vi "Master-vi_v1_9_0.vi"() -> ()   [LabVIEW 2024]
uses:
  QMH-Architecture/UI-Controls/UI State.ctl
  QMH-Architecture/support/Control/Waveform Data Constant.ctl
  QMH-Architecture/support/Control/Array Data Constant.ctl
  QMH-Architecture/Aborts/Abort Parameters.ctl
  QMH-Architecture/support/Control/Control Data Constant.ctl
  QMH-Architecture/Sequence/Sequence Structure.ctl
  QMH-Architecture/support/Control/BBControl Parameters.ctl
  QMH-Architecture/Display/Global 1.vi
  <vilib>/Utility/error.llb/Error Cluster From Error Code.vi
  QMH-Architecture/Globals.vi
  <vilib>/ErrorRing/Error Ring.xnode
  QMH-Architecture/support/User Event - Stop/User Event - Stop.lvlib
  QMH-Architecture/support/Message Queue/Message Queue.lvlib
panel:
  out "Total Physical Memory":u64 format="%.1p"
  out "Memory Allocated For LabVIEW":u64 format="%.1p"
  out "Free Physical Memory":u64 format="%.1p"
  out "UI Elements":i32
  out "Acquisition Elements":i32
  out "Logging Elements":i32
  out "Controls Elements":i32
  out "Sequence Elements":i32
  out "Aborts Elements":i32
  out "Processed Data":i32
  out "Unprocessed Data":i32
  out "Controls Iteration Clock":u32
  out "Acquisition Iteration Clock":u32
  out "Processing_Logging Iteration Clock":u32
  out "Sequencing Iteration Clock":u32
  out "Aborts Iteration Clock":u32
  in  "System Monitor":bool
  in  "Control Monitor":bool
  out "Network Stream Clock":u32
  out "NetworkStream Elements":i32
  out "Waveform Chart":i16[](graph)
  in  "Graph Display":bool
  out "Status":T1(array[cluster]) {"Status Timestamp" format="%<%H:%M:%S%3u>T"}
  out "Timestamp":timestamp format="%<%H:%M:%S%3u>T"
  in  "Load Name":bool
  in  "File name":string
  out "Display-Loop Iteration Clock (ms)":u32
  in  "Status clear":bool
  out "Logging Status":bool
  in  "Exit Button":bool
  in  "Stop Button":bool
  in  "Data log":bool
  # "User Interface"
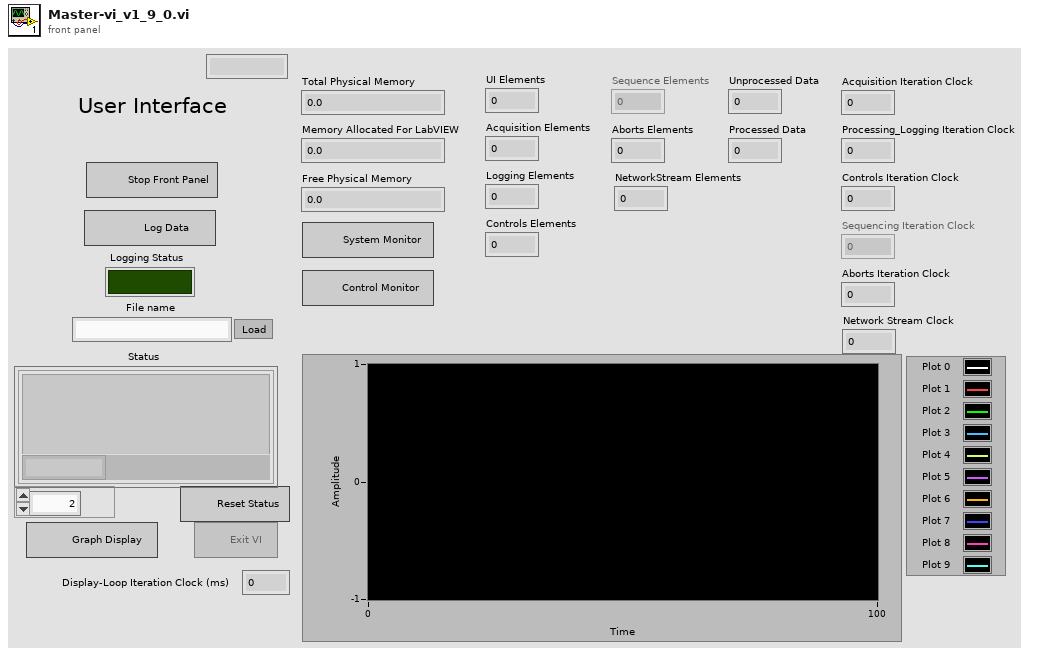
[diagram p1: front panel]
types:
  T1 = cluster{"Status":string, "Status Timestamp":timestamp}[]
  T2 = typedef "BBControl Parameters.ctl" = cluster{"Sequence Delay (s)":dbl, "Sequence Duration (s)":dbl, "BBControl Criteria":cluster{"Channel Name":i32, "Comparison":u16, "Set":dbl, "Enabled":bool, "Valve Name":i32, "Upper":dbl, "Lower":dbl}[]}
  T3 = typedef "Sequence Structure.ctl" = cluster{"Sequence Controller":cluster{"Time (s)":dbl, "Enabled":bool, "Valve":u16[]}[], "Sequence Delay":dbl, "Sequence Duration":dbl}
  T4 = typedef "Control Data Constant.ctl" = cluster{"Time (utc)":ext, "Data Out":cluster{"DO":bool[], "Module Number":string}[]}
  T5 = typedef "Abort Parameters.ctl" = cluster{"Sequence Delay (s)":dbl, "Sequence Duration (s)":dbl, "Abort Criteria":cluster{"Channel Name\n":enum16{"[0]", "[1]", "[2]", "[3]", "[4]", "[5]", "[6]", "[7]", "[8]", "[9]", "[10]", "[11]", "[12]", "[13]", "[14]", "[15]", "[16]", "[17]", "[18]", "[19]", "[20]", "[21]", "[22]", "[23]", "[24]", "[25]", "[26]", "[27]", "[28]", "[29]", "[30]", "[31]", "[32]", "[33]", "[34]", "[35]", "[36]", "[37]", "[38]", "[39]", "[40]", "[41]", "[42]", "[43]", "[44]", "[45]", "[46]", "[47]", "[48]", "[49]"}, "Comparison\n":u16, "Threshold":dbl, "Time on (s)":dbl, "Time off (s)":dbl, "Enabled":bool}[]}
  T6 = typedef "Array Data Constant.ctl" = cluster{"AI":dbl[], "TC":dbl[], "BC":dbl[], "DI":dbl[], "t (UTC)":dbl}
  T7 = typedef "Waveform Data Constant.ctl" = cluster{"AI":waveform(dbl)[], "TC":waveform(dbl)[], "BC":waveform(dbl)[], "DI":digitalwaveform[], "DI2":digitalwaveform[]}
  T8 = typedef "UI State.ctl" = enum16{"Idle", "Acquiring", "Logging", "Waiting for Exit", "Waiting for Exit (Acq Stopped)", "Waiting for Exit (Log Stopped)", "Waiting for Stop", "Waiting for Stop (Acq Stopped)", "Waiting for Stop (Log Stopped)"}
  T9 = typedef "Message Queue.lvlib/All Message Queues.ctl" = cluster{"UI":refnum<queue>, "Acquisition":refnum<queue>, "Logging":refnum<queue>, "Controls":refnum<queue>, "Sequence":refnum<queue>, "Aborts":refnum<queue>, "Network Streams":refnum<queue>}
  T10 = cluster{"Status":string, "Status Timestamp":timestamp}
  T11 = typedef "DAQmx Configuration.ctl" = cluster{"ai DAQmx Cluster":cluster{"ai PXIe Task Name":string[], "input terminal configuration":i32[]}, "bc DAQmx Cluster":cluster{"bc PXIe Task Name":string[], "Scaling Information":cluster{"first electrical value":dbl, "second electrical value":dbl, "electrical units":i32, "first physical value":dbl, "second physical value":dbl, "physical units":i32}[], "Bridge Information":cluster{"bridge configuration":i32, "voltage excitation source":i32, "voltage excitation value":dbl, "nominal bridge resistance":dbl}[]}, "tc DAQmx Cluster":cluster{"tc PXIe Task Name":string[], "Thermocouple Type":i32[], "Units":i32[]}, "di DAQmx Cluster":cluster{"di PXIe Task Name":string[]}, "do DAQmx Cluster":cluster{"do PXIe Task Name":string[]}, "ao DAQmx Cluster":cluster{"ao PXIe Task Name":string[]}}
  T12 = typedef "StreamCluster_TypeDef.ctl" = cluster{"DAQ":cluster{"ManagmentRate_Hz":i32, "StreamRate_Hz":i32, "StreamRate_ms":i32, "ManagmentRate_ms":i32, "refDesArray":cluster{"refDes-s":string[], "Module Number":string}[]}, "Modules":cluster{"Slot ID":i32, "Model Number":string, "Sample Rate s/S (Hz)":dbl, "Sensors":cluster{"refDes":string, "serialNumber":string, "modelNumber":string, "units":string, "balance":dbl, "sensitivity":dbl, "type":string, "inputTerminalConfiguration":string, "channelNumber":string, "taskName":string, "bridgeConfiguration":string, "excitationVoltage":dbl, "voltageExcitationSource":string, "nominalBridgeResistance":dbl, "firstElectricalValue":dbl, "secondElectricalValue":dbl, "firstPhysicalValue":dbl, "secondPhysicalValue":dbl, "electricalUnits":string}[]}[]}
  T13 = typedef "Calibration Configuration.ctl" = cluster{"ai Calibration Slope":dbl[], "ai Calibration Offset":dbl[], "ai Sensor Names ":string[], "tc Sensor Names":string[], "di Sensor Names":string[], "do Sensor Names":string[], "bc Sensor Names":string[], "ai Sensor Units":string[], "tc Sensor Units":string[], "bc Sensor Units":string[]}
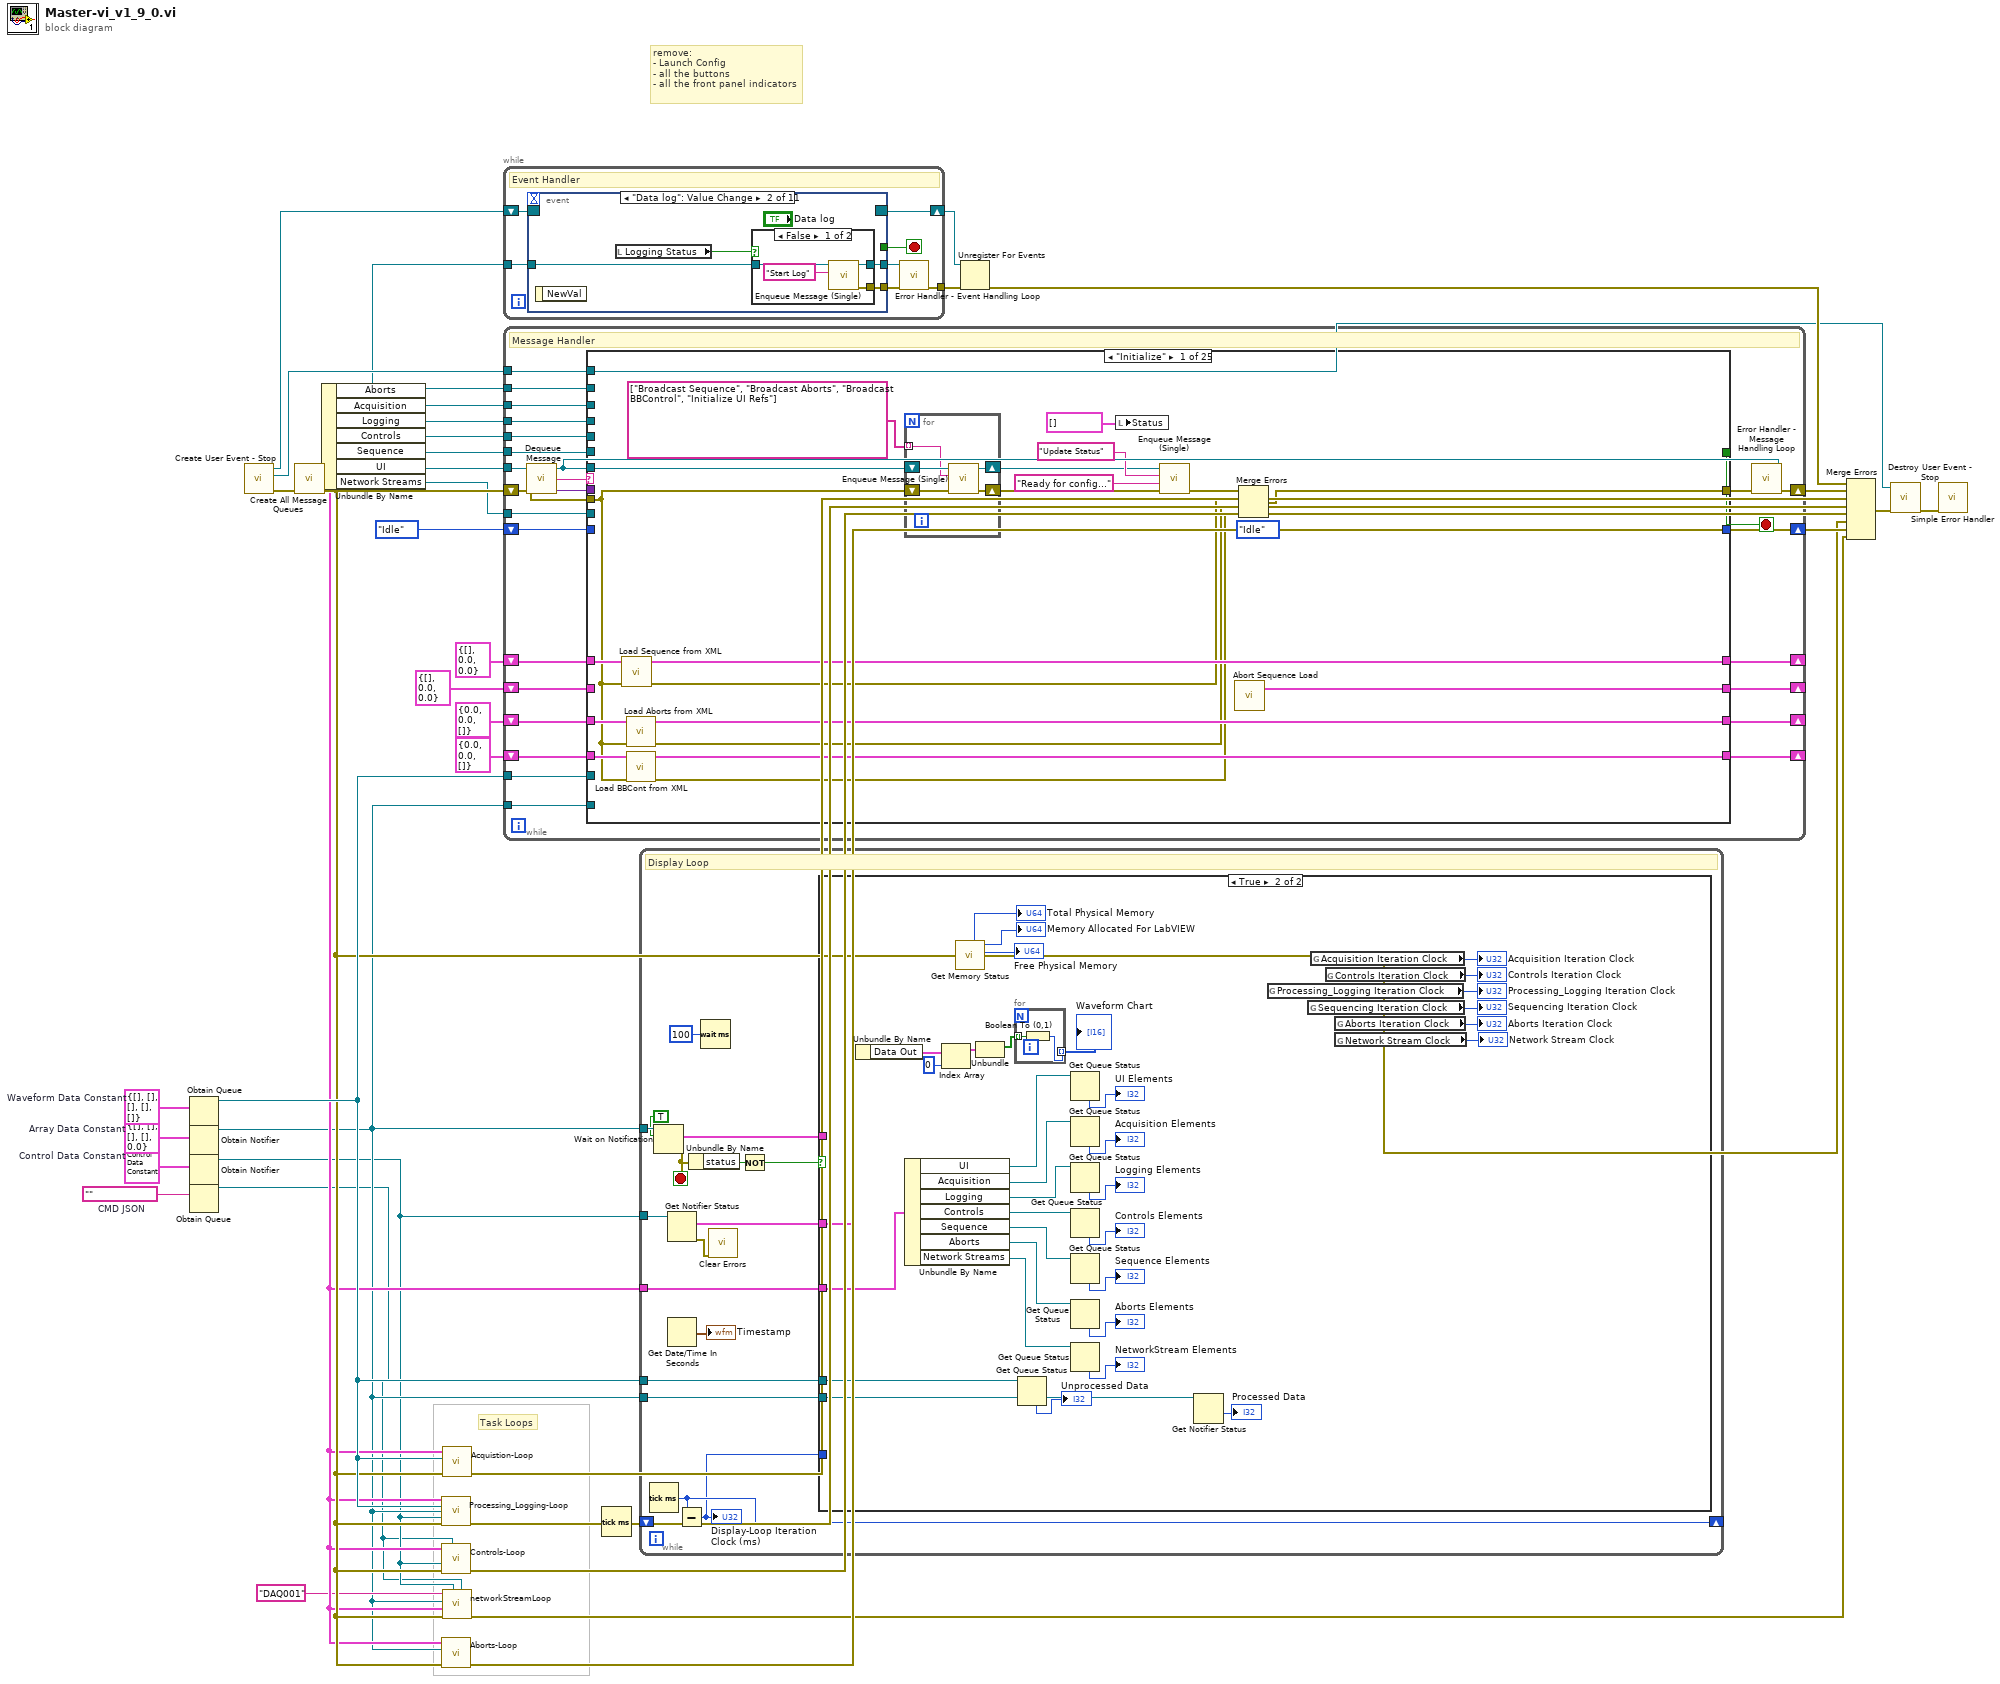
[diagram p0: block diagram]
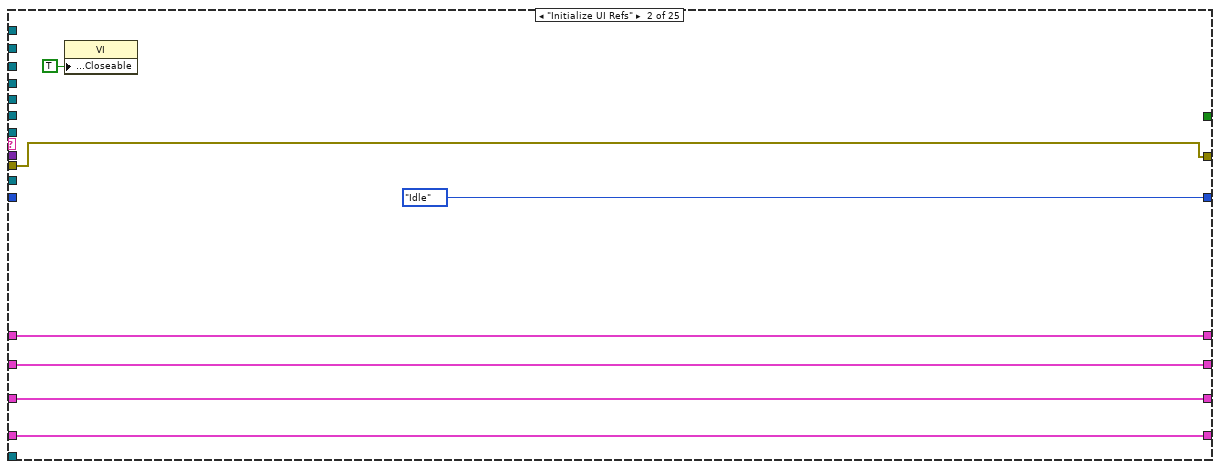
[diagram p3: hidden frame]
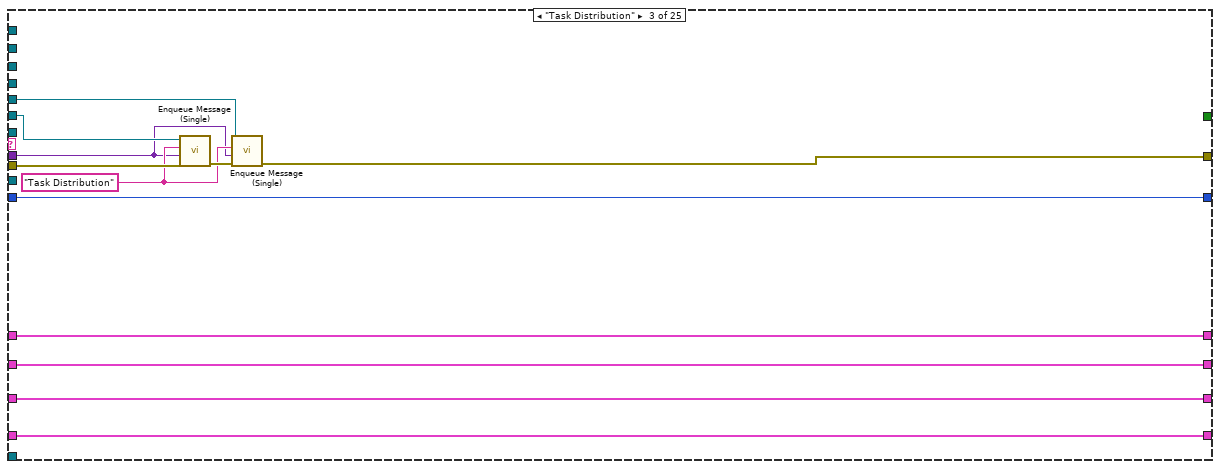
[diagram p4: hidden frame]
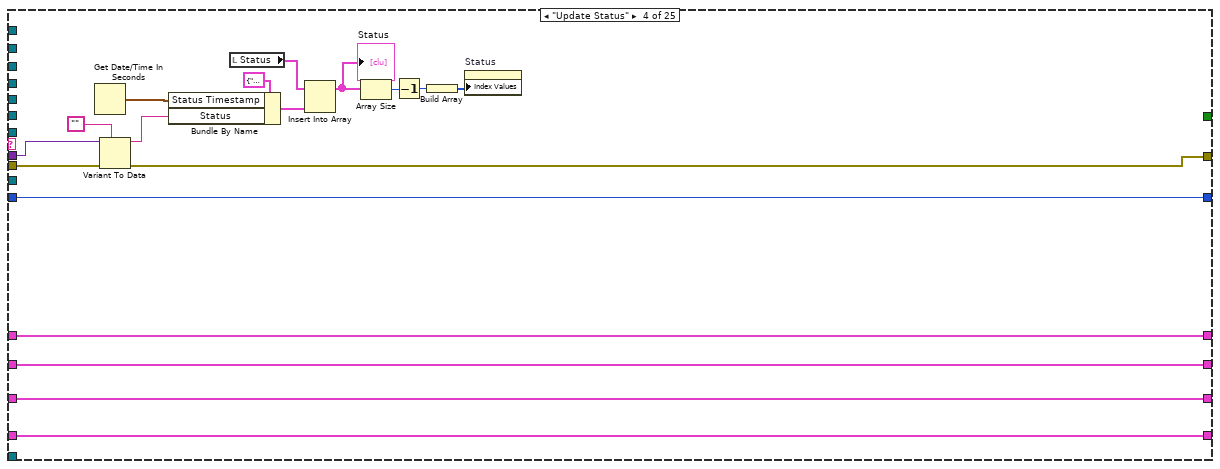
[diagram p5: hidden frame]
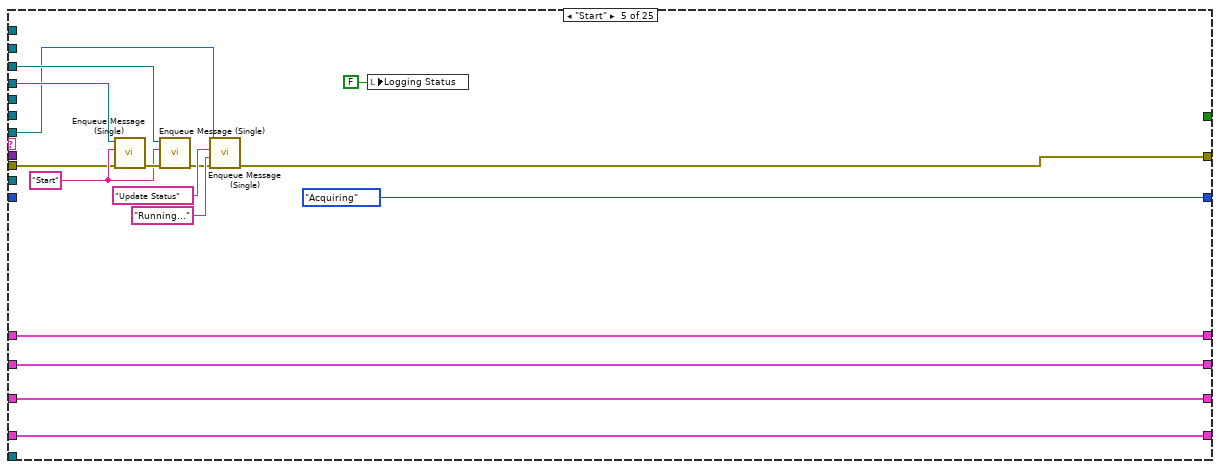
[diagram p6: hidden frame]
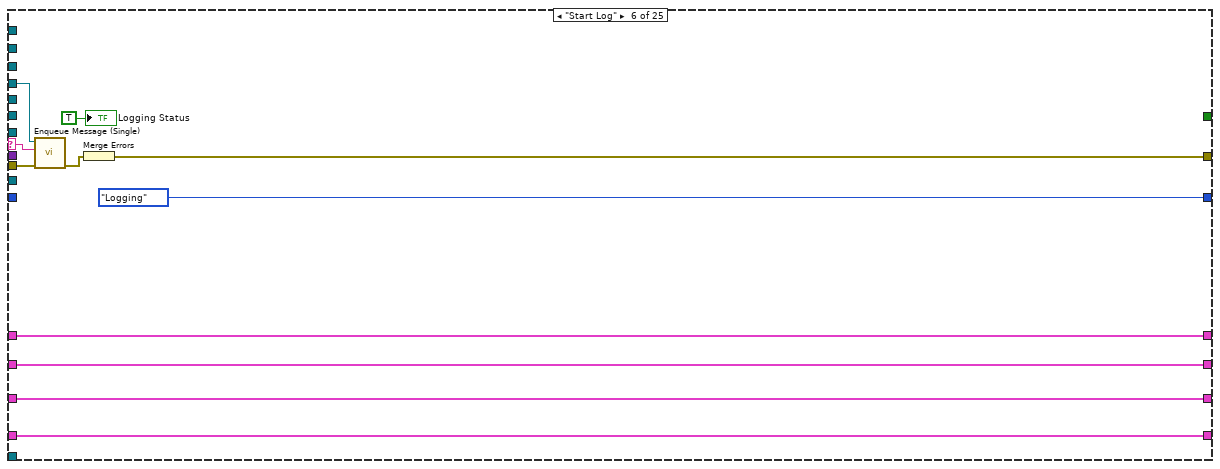
[diagram p7: hidden frame]
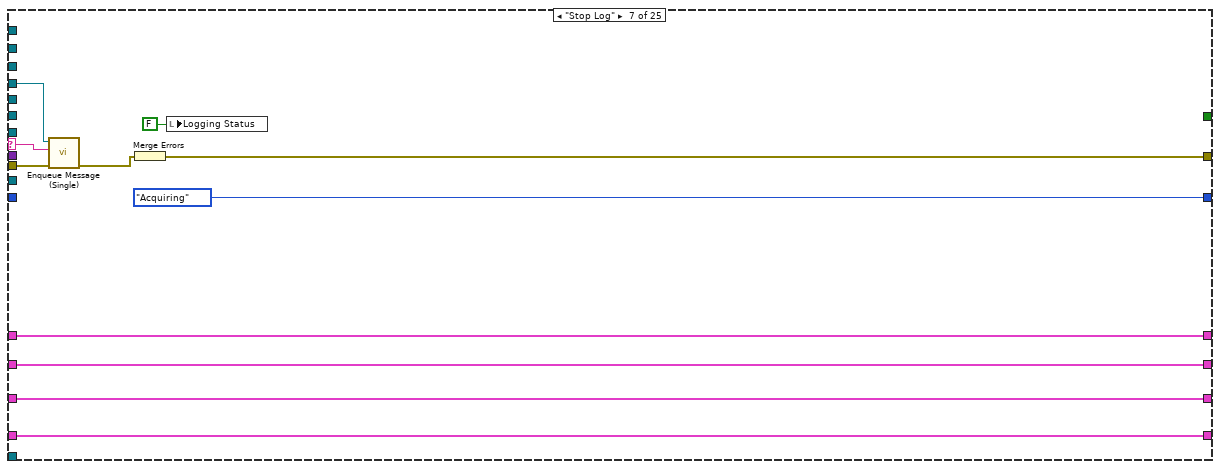
[diagram p8: hidden frame]
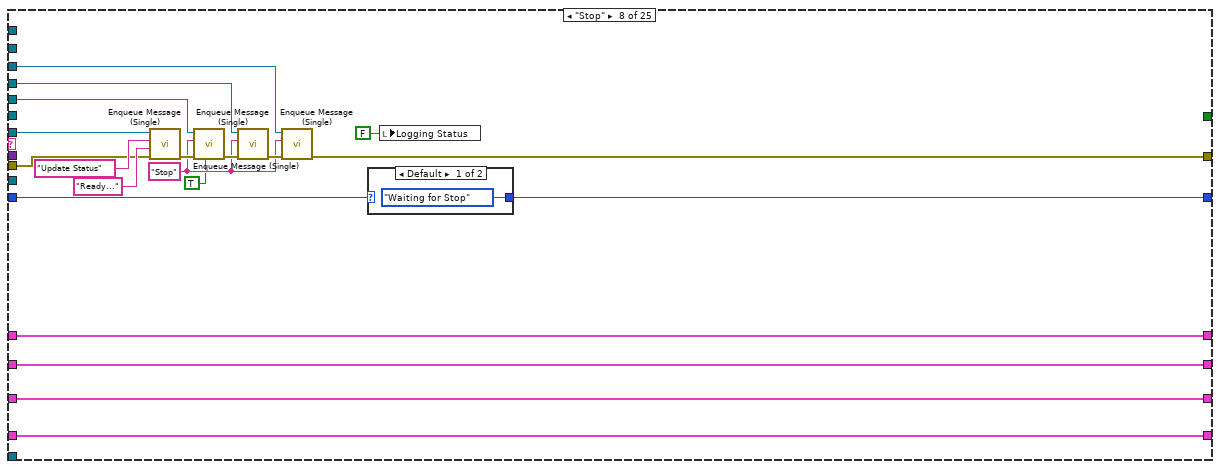
[diagram p9: hidden frame]
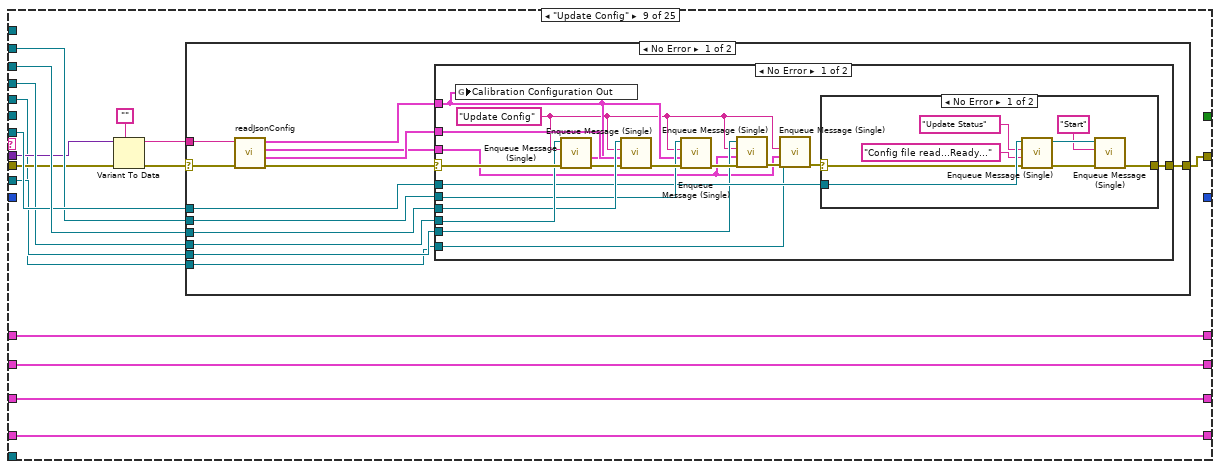
[diagram p11: hidden frame]
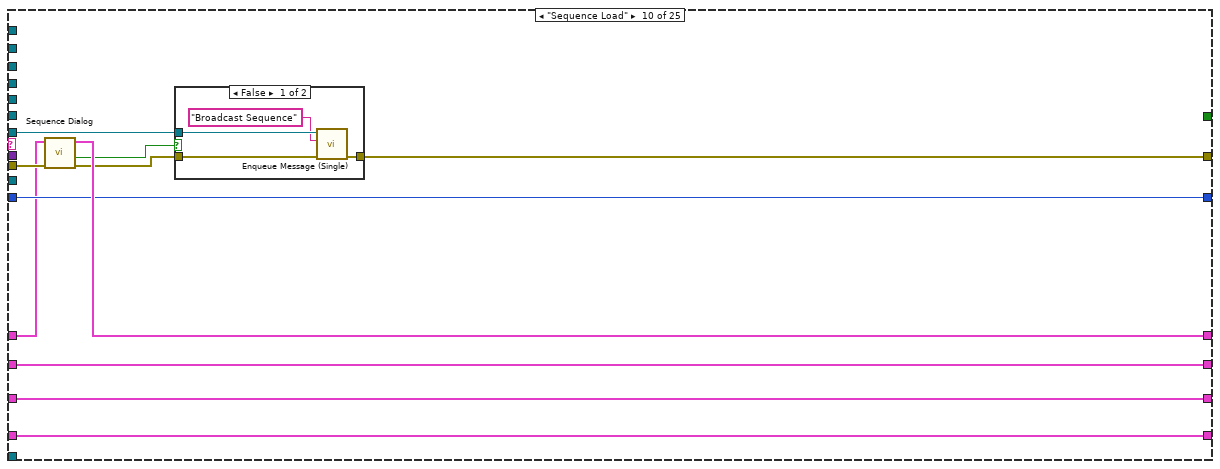
[diagram p15: hidden frame]
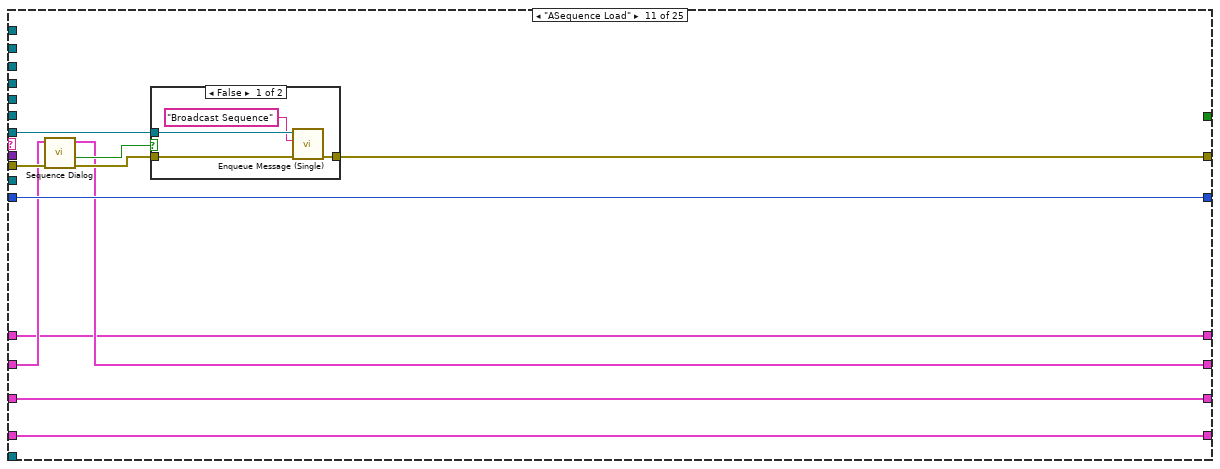
[diagram p17: hidden frame]
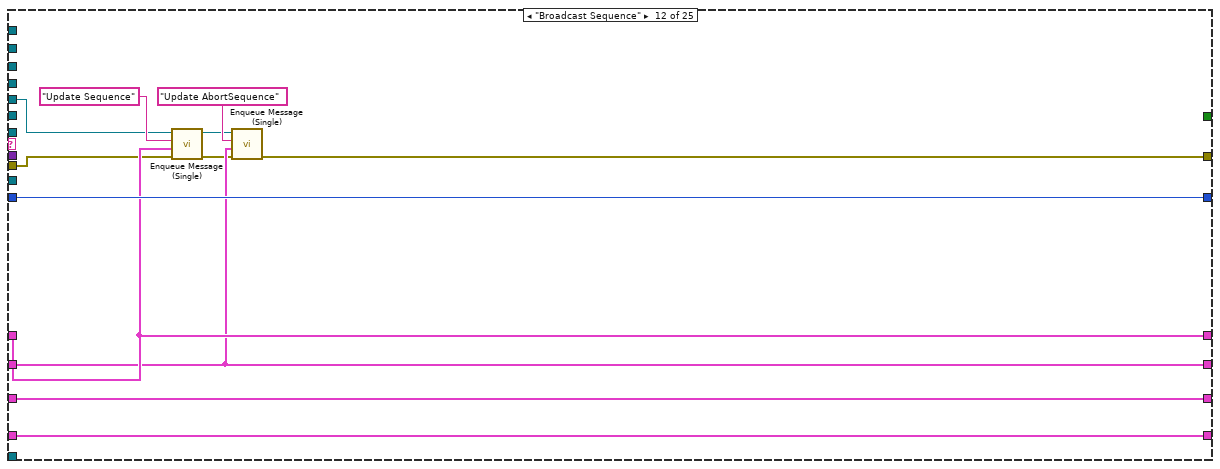
[diagram p19: hidden frame]
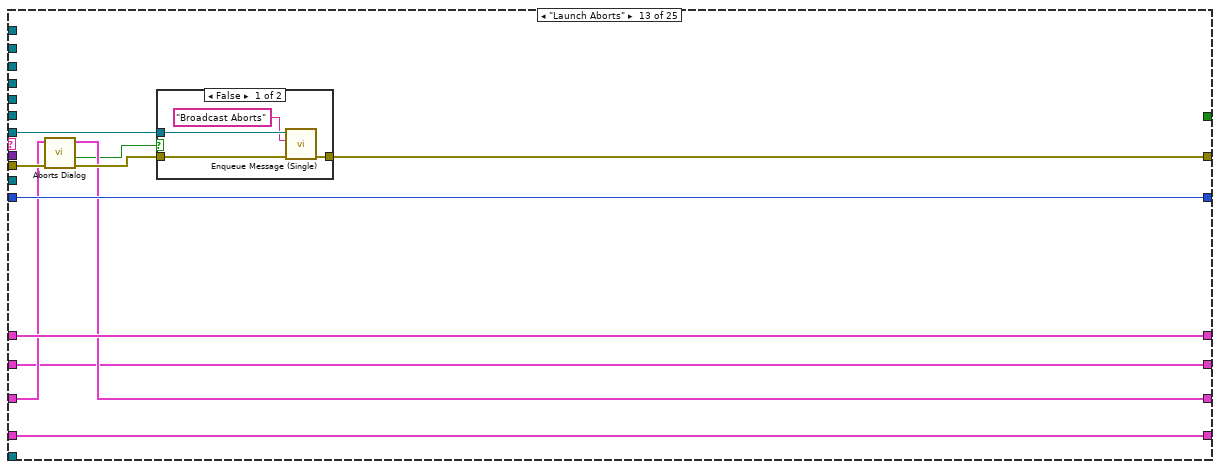
[diagram p20: hidden frame]
diagram:
  w2 = ""  # CMD JSON
  w12 = T4 {"Time (utc)"=0.0, "Data Out"=[]}  # Control Data Constant
  w19 = T6 {"AI"=[], "TC"=[], "BC"=[], "DI"=[], "t (UTC)"=0.0}  # Array Data Constant
  w20 = T7 {"AI"=[], "TC"=[], "BC"=[], "DI"=[], "DI2"=[]}  # Waveform Data Constant
  # "remove:\n- Launch Config\n- all the buttons\n- all the front panel indicators"
  # "Task Loops"
  n1 = Obtain Queue(element data type=w20) -> (queue out=w13:refnum<queue>)  [unwired: 4 in, 2 out]
  n2 = Obtain Notifier(notification data type=w19) -> (notifier out=w4:refnum<notifier>)  [unwired: 3 in, 2 out]
  n3 = Obtain Notifier(notification data type=w12) -> (notifier out=w3:refnum<notifier>)  [unwired: 3 in, 2 out]
  n4 = Obtain Queue(element data type=w2) -> (queue out=w1:refnum<queue>)  [unwired: 4 in, 2 out]
  n5 = call "Create User Event - Stop.vi"() -> ("error out"=w35:errorcluster, "User Event - Stop"=w28:refnum<user-event>, "Stop Event Registration Refnum"=w38:refnum<event-registration>)  [unwired: 9 in]
  n6 = call "Create All Message Queues.vi"("error in (no error)"=w35) -> ("error out"=w9:errorcluster, "Message Queues out"=w6:T9)  [unwired: 9 in]
  n7 = Unbundle By Name(w6) -> ("Aborts"=w27:refnum<queue>, "Acquisition"=w32:refnum<queue>, "Logging"=w31:refnum<queue>, "Controls"=w30:refnum<queue>, "Sequence"=w29:refnum<queue>, "UI"=w26:refnum<queue>, "Network Streams"=w7:refnum<queue>)
  n8 = call "Processing_Logging-Loop.vi"("Message Queues"=w6, "Unprocessed Data"=w13, "Processed Data Notifier"=w4, "Control Data Notifier"=w3, "error in"=w9) -> ("error out"=w23:errorcluster)  [unwired: 10 in]
  n9 = call "Controls-Loop.vi"("JSON cmd queue"=w1, "error in"=w9, "Control Data Notifier"=w3, "Message Queues"=w6) -> ("error out"=w21:errorcluster)  [unwired: 7 in]
  n10 = call "Aborts-Loop.vi"("Message Queues"=w6, "Processed Data Notifier"=w4, "error in"=w9) -> ("error out"=w18:errorcluster)  [unwired: 7 in]
  n11 = call "Acquistion-Loop.vi"("error in"=w9, "Unprocessed Data"=w13, "Message Queues"=w6) -> ("error out"=w24:errorcluster)  [unwired: 8 in]
  n12 = call "networkStreamLoop.vi"("JSON cmd queue"=w1, "Control Data Notifier"=w3, "error in"=w9, "Message Queues"=w6, "Processed Data Notifier"=w4, "daqRefDes"="DAQ001" ("DAQ Endpoint")) -> ("error out"=w8:errorcluster)  [unwired: 5 in]
  n13 = while {
    shift-right: [w44] -> w36
    shift-left: w38 -> [w45]
    tunnel: [w43] -> w37
    tunnel: w26 -> [w41]
    stop <- w40 stop-if-true
    # "Event Handler"
    n14 = event shown="[1] \"Data log\": Value Change" {
      selector: w45 -> [_ _ _ _ _ _ _ _ _ _ _]
      dyn-events: [_ _ _ _ _ _ _ _ _ _ _] -> w44
      timeout: _ -> [_ _ _ _ _ _ _ _ _ _ _]
      tunnel: [w48 w53 w68 w71 w75 w79 w84 w88 w95 w96 w97] -> w42
      tunnel: w41 -> [w47 w51 w64 w70 w74 w78 w85 w86 w94 w96 w97]
      tunnel: [_ _ _ _ _ _ _ _ _ _ TRUE] -> w40
      tunnel: [w49 w52 w67 w72 w76 w80 w83 w87 w91 _ _] -> w39
      event "Stop Button": Value Change {
        n15 = event-data() -> ()  [unwired: 1 in, 1 out]
        n16 = call "Enqueue Message (Single).vi"("Message"="Stop", "Message Queue"=w47) -> ("error out"=w49:errorcluster, "dup Message Queue"=w48:refnum<queue>)  [unwired: 8 in]
      }
      event "Data log": Value Change {
        n17 = event-data() -> ()  [unwired: 1 in, 1 out]
        n18 = local read "Logging Status"() -> (w50:bool)
        n19 = case shown="False" w50 {
          tunnel: [w57 w61] -> w53
          tunnel: [w56 w60] -> w52
          tunnel: w51 -> [w55 w59]
          frame False {
            n20 = call "Enqueue Message (Single).vi"("Message"="Start Log", "Message Queue"=w55) -> ("error out"=w56:errorcluster, "dup Message Queue"=w57:refnum<queue>)  [unwired: 8 in]
          }
          frame True {
            n21 = call "Enqueue Message (Single).vi"("Message Data"="Ready...", "Message"="Stop Log", "Message Queue"=w59) -> ("error out"=w60:errorcluster, "dup Message Queue"=w61:refnum<queue>)  [unwired: 7 in]
          }
        }
      }
      event "Status clear": Value Change {
        n22 = event-data() -> ()  [unwired: 1 in, 1 out]
        n23 = call "Enqueue Message (Single).vi"("Message Data"="Ready...", "Message"="Update Status", "Message Queue"=w64) -> ("error out"=w67:errorcluster, "dup Message Queue"=w68:refnum<queue>)  [unwired: 7 in]
        n24 = local write "Status"(T1 [] ("Status 1")) -> ()
      }
      event "System Monitor": Value Change {
        n25 = event-data() -> ()  [unwired: 1 in, 1 out]
        n26 = call "Enqueue Message (Single).vi"("Message"="System Monitor", "Message Queue"=w70) -> ("error out"=w72:errorcluster, "dup Message Queue"=w71:refnum<queue>)  [unwired: 8 in]
      }
      event "Control Monitor": Value Change {
        n27 = event-data() -> ()  [unwired: 1 in, 1 out]
        n28 = call "Enqueue Message (Single).vi"("Message"="Control Monitor", "Message Queue"=w74) -> ("error out"=w76:errorcluster, "dup Message Queue"=w75:refnum<queue>)  [unwired: 8 in]
      }
      event "Graph Display": Value Change {
        n29 = event-data() -> ()  [unwired: 1 in, 1 out]
        n30 = call "Enqueue Message (Single).vi"("Message"="Graph Display", "Message Queue"=w78) -> ("error out"=w80:errorcluster, "dup Message Queue"=w79:refnum<queue>)  [unwired: 8 in]
      }
      event "Load Name": Value Change {
        n31 = event-data() -> ()  [unwired: 1 in, 1 out]
        n32 = call "Enqueue Message (Single).vi"("Message Data"="File name", "Message"="Load File Name", "Message Queue"=w85) -> ("error out"=w83:errorcluster, "dup Message Queue"=w84:refnum<queue>)  [unwired: 7 in]
      }
      event "Exit Button": Value Change; Panel Close {
        n33 = event-data() -> ()  [unwired: 1 in, 1 out]
        n34 = call "Enqueue Message (Single).vi"("Priority Message? (F)"=TRUE, "Message"="Leave", "Message Queue"=w86) -> ("error out"=w87:errorcluster, "dup Message Queue"=w88:refnum<queue>)  [unwired: 7 in]
      }
      event Panel Close? {
        w92 = TRUE ("Priority Message? (F)")
        n35 = event-data() -> ()  [unwired: 1 in, 1 out]
        n36 = call "Enqueue Message (Single).vi"("Priority Message? (F)"=w92, "Message"="Confirm Quit", "Message Queue"=w94) -> ("error out"=w91:errorcluster, "dup Message Queue"=w95:refnum<queue>)  [unwired: 7 in]
        n37 = event-data("Discard?"=w92) -> ()  [unwired: 1 in, 1 out]
      }
      event Application Instance Close {
        n38 = event-data() -> ()  [unwired: 1 in, 1 out]
      }
      event User Event {
        n39 = event-data() -> ()  [unwired: 1 in, 1 out]
      }
    }
    n40 = call "Error Handler - Event Handling Loop.vi"("error in (no error)"=w39, "Message Queue"=w42) -> ("dup error in"=w43:errorcluster)  [unwired: 8 in, 1 out]
  }
  n41 = while {
    shift-right: [w126] -> w33
    shift-left: w9 -> [w125]
    tunnel: w27 -> [w120]
    tunnel: w32 -> [w121]
    tunnel: w31 -> [w122]
    tunnel: w30 -> [w123]
    tunnel: w29 -> [w103]
    tunnel: w26 -> [w124]
    tunnel: w28 -> [w119]
    shift-right: [w112] -> _
    shift-left: UI_State."Idle" ("UI State") -> [w113]
    tunnel: w13 -> [w109]
    tunnel: w4 -> [w110]
    shift-right: [w99] -> _
    shift-left: T3 {"Sequence Controller"=[], "Sequence Delay"=0.0, "Sequence Duration"=0.0} ("Sequence Conditions") -> [w108]
    shift-right: [w106] -> _
    shift-left: T5 {"Sequence Delay (s)"=0.0, "Sequence Duration (s)"=0.0, "Abort Criteria"=[]} ("Abort Parameters") -> [w107]
    shift-right: [w104] -> _
    shift-left: T3 {"Sequence Controller"=[], "Sequence Delay"=0.0, "Sequence Duration"=0.0} ("Sequence Conditions") -> [w105]
    shift-right: [w101] -> _
    shift-left: T2 {"Sequence Delay (s)"=0.0, "Sequence Duration (s)"=0.0, "BBControl Criteria"=[]} ("BangBang Valve Control") -> [w102]
    tunnel: w7 -> [w100]
    stop <- w111 stop-if-true
    # "Message Handler"
    n42 = call "Dequeue Message.vi"("error in (no error)"=w125, "Message Queue"=w124) -> ("error out"=w115:errorcluster, "Message Data"=w116:variant, "Message"=w117:string, "dup Message Queue"=w118:refnum<queue>)  [unwired: 6 in]
    n43 = case "Message Cases" shown="\"Initialize\"" w117 {
      selector: w117 -> [_ _ _ _ _ w215 w225 _ _ _ _ _ _ _ _ _ w403 _ _ _ _ _ _ _ w523]
      tunnel: w118 -> [w129 _ _ _ w195 _ _ w239 w259 w314 w331 _ w360 _ w385 _ _ _ _ _ _ _ w468 w508 _]
      tunnel: w103 -> [_ _ w166 _ _ _ _ _ _ _ _ _ _ _ _ _ _ _ _ _ _ _ _ w510 _]
      tunnel: w123 -> [_ _ w165 _ _ _ _ w237 w250 _ _ w340 _ _ _ w392 _ _ _ _ _ _ _ w509 _]
      tunnel: w122 -> [_ _ _ _ w203 w214 w227 w236 w257 _ _ _ _ _ _ _ w405 _ _ _ _ _ _ w511 _]
      tunnel: w121 -> [_ _ _ _ w202 _ _ w235 w262 _ _ _ _ _ _ _ _ _ _ _ _ _ _ w512 _]
      tunnel: w120 -> [_ _ _ _ _ _ _ _ w258 _ _ _ _ w372 _ _ _ _ _ _ _ _ _ w513 _]
      tunnel: w119 -> [_ _ _ _ _ _ _ _ _ _ _ _ _ _ _ _ _ _ _ _ _ _ _ w514 _]
      tunnel: w116 -> [_ _ w162 w188 _ _ _ _ w253 _ _ _ _ _ _ _ w404 _ _ _ _ w461 _ _ _]
      tunnel: w115 -> [w128 w155 w168 w187 w194 w209 w220 w238 w256 w313 w330 w346 w357 w373 w382 w398 w410 w414 w421 w429 w439 w457 w469 w499 _]
      tunnel: [w141 w155 w163 w185 w192 w216 w226 w229 w263 w315 w332 w342 w359 w370 w384 w396 w406 w413 w420 w428 w437 w462 w467 w507 w524] -> w114
      tunnel: w113 -> [_ _ w171 w189 _ _ _ w247 _ w316 w333 w350 w361 w374 w386 w399 w409 w415 w423 w431 w446 w456 w471 _ w525]
      tunnel: [UI_State."Idle" ("UI State") UI_State."Idle" ("UI State") w171 w189 UI_State."Acquiring" ("UI State") UI_State."Logging" ("UI State") UI_State."Acquiring" ("UI State") w246 _ w316 w333 w350 w361 w374 w386 w399 w409 w415 w423 w431 w446 w456 w470 UI_State."Idle" ("UI State") w525] -> w112
      tunnel: [_ _ _ _ _ _ _ _ _ _ _ _ _ _ _ _ _ _ _ _ _ _ _ TRUE _] -> w111
      tunnel: w110 -> [_ _ _ _ _ _ _ _ _ _ _ _ _ _ _ _ _ _ _ _ w435 _ _ w504 _]
      tunnel: w109 -> [_ _ _ _ _ _ _ _ _ _ _ _ _ _ _ _ _ _ _ _ _ _ _ w503 _]
      tunnel: w108 -> [w140 w157 w170 w184 w198 w212 w223 w234 w265 w310 w324 w348 w358 w375 w383 w400 w408 w416 w424 w432 w447 w459 w466 w517 w522]
      tunnel: [w139 w157 w170 w184 w198 w212 w223 w234 w265 w317 w324 w348 w358 w375 w383 w400 w408 w416 w424 w432 w447 w459 w466 w517 w522] -> w99
      tunnel: w107 -> [w144 w156 w169 w183 w197 w211 w222 w233 w264 w309 w327 w347 w355 w369 w377 w395 w407 w417 w425 w433 w448 w458 w465 w518 w521]
      tunnel: [w143 w156 w169 w183 w197 w211 w222 w233 w264 w309 w327 w347 w354 w369 w377 w395 w407 w417 w425 w433 w448 w458 w465 w518 w521] -> w106
      tunnel: w105 -> [_ w154 w161 w173 w193 w210 w221 w231 w261 w308 w326 w344 w352 w368 w379 w394 w402 w412 w419 w427 w445 w455 w464 w497 w520]
      tunnel: [w133 w154 w161 w173 w193 w210 w221 w231 w261 w308 w325 w344 w352 w368 w379 w394 w402 w412 w419 w427 w445 w455 w464 w497 w520] -> w104
      tunnel: w102 -> [w131 w153 w160 w172 w190 w206 w217 w228 w260 w307 w323 w339 w351 w367 w378 w393 w401 w411 w418 w426 w434 w454 w463 w496 w519]
      tunnel: [w132 w153 w160 w172 w190 w206 w217 w228 w260 w307 w323 w339 w351 w367 w376 w393 w401 w411 w418 w426 w434 w454 w463 w496 w519] -> w101
      tunnel: w100 -> [_ _ _ _ _ _ _ _ w251 _ _ _ _ _ _ _ _ _ _ _ _ w450 _ w495 _]
      frame "Initialize" {
        n44 = call "Load Sequence from XML.vi"("error in (no error)"=w128, "Sequence Conditions In"=w140) -> ("error out"=w137:errorcluster, "Sequence Conditions Out"=w139:T3)  [unwired: 8 in]
        n45 = call "Load Aborts from XML.vi"("error in (no error)"=w128, "Abort Parameters In"=w144) -> ("error out"=w138:errorcluster, "Abort Parameters Out"=w143:T5)  [unwired: 8 in]
        n46 = call "Load BBCont from XML.vi"("error in (no error)"=w128, "BBCont Parameters In"=w131) -> ("error out"=w130:errorcluster, "BBCont Parameters Out"=w132:T2)  [unwired: 8 in]
        n47 = for {
          shift-right: [w151] -> w135
          shift-left: w129 -> [w150]
          shift-right: [w152] -> w136
          shift-left: w128 -> [w149]
          tunnel: string[] ["Broadcast Sequence", "Broadcast Aborts", "Broadcast BBControl", "Initialize UI Refs"] -> [w148] mode=indexing
          n48 = call "Enqueue Message (Single).vi"("error in (no error)"=w149, "Message"=w148, "Message Queue"=w150) -> ("error out"=w152:errorcluster, "dup Message Queue"=w151:refnum<queue>)  [unwired: 7 in]
        }
        n49 = local write "Status"(T1 [] ("Status 1")) -> ()
        n50 = call "Enqueue Message (Single).vi"("error in (no error)"=w136, "Message Data"="Ready for config...", "Message"="Update Status", "Message Queue"=w135) -> ("error out"=w142:errorcluster)  [unwired: 6 in, 1 out]
        n51 = call "Abort Sequence Load.vi"() -> ("Abort Sequence"=w133:T3)  [unwired: 3 in]
        n52 = Merge Errors(w142, w137, w138, w130) -> (w141:errorcluster)
      }
      frame "Initialize UI Refs" {
        n53 = property class="VI"("Front Panel.Closeable"=TRUE) -> ()  [unwired: 2 in, 2 out]
      }
      frame "Task Distribution" {
        w164 = "Task Distribution"
        n54 = call "Enqueue Message (Single).vi"("error in (no error)"=w168, "Message Data"=w162, "Message"=w164, "Message Queue"=w166) -> ("error out"=w167:errorcluster)  [unwired: 6 in, 1 out]
        n55 = call "Enqueue Message (Single).vi"("error in (no error)"=w167, "Message Data"=w162, "Message"=w164, "Message Queue"=w165) -> ("error out"=w163:errorcluster)  [unwired: 6 in, 1 out]
      }
      frame "Update Status" {
        n56 = Get Date/Time In Seconds() -> (seconds since 1Jan1904=w180:timestamp)
        n57 = Variant To Data(error in=w187, type="", Variant=w188) -> (data=w179:string, error out=w185:errorcluster)
        n58 = Bundle By Name(cluster=T10 {"Status"="", "Status Timestamp"=timestamp(0 s since 1904-01-01)} ("Cluster"), "Status Timestamp"=w180, "Status"=w179) -> (w181:T10)
        n59 = local read "Status"() -> (w175:T1)
        n60 = Insert Into Array(array=w175, new element=w181) -> (w177:T1)  [unwired: 1 in]
        "Status" <- w177
        n61 = Array Size(array=w177) -> (size(s)=w176:i32)
        n62 = Decrement(x=w176) -> (x-1=w174:i32)
        n63 = Build Array(w174) -> (w178:i32[])
        n64 = property on="Status" class="Arr (strict)"("Index Values"=w178) -> ()  [unwired: 2 in, 2 out]
      }
      frame "Start" {
        w201 = "Start"
        n65 = call "Enqueue Message (Single).vi"("error in (no error)"=w194, "Message"=w201, "Message Queue"=w203) -> ("error out"=w204:errorcluster)  [unwired: 7 in, 1 out]
        n66 = call "Enqueue Message (Single).vi"("error in (no error)"=w204, "Message"=w201, "Message Queue"=w202) -> ("error out"=w196:errorcluster)  [unwired: 7 in, 1 out]
        n67 = call "Enqueue Message (Single).vi"("error in (no error)"=w196, "Message Data"="Running...", "Message"="Update Status", "Message Queue"=w195) -> ("error out"=w192:errorcluster)  [unwired: 6 in, 1 out]
        n68 = local write "Logging Status"(FALSE ("Logging Status")) -> ()
      }
      frame "Start Log" {
        n69 = call "Enqueue Message (Single).vi"("error in (no error)"=w209, "Message"=w215, "Message Queue"=w214) -> ("error out"=w213:errorcluster)  [unwired: 7 in, 1 out]
        n70 = Merge Errors(w213) -> (w216:errorcluster)
        "Logging Status" <- TRUE ("Logging Status")
      }
      frame "Stop Log" {
        n71 = call "Enqueue Message (Single).vi"("error in (no error)"=w220, "Message"=w225, "Message Queue"=w227) -> ("error out"=w224:errorcluster)  [unwired: 7 in, 1 out]
        n72 = Merge Errors(w224) -> (w226:errorcluster)
        n73 = local write "Logging Status"(FALSE ("Logging Status")) -> ()
      }
      frame "Stop" {
        w242 = "Stop"
        n74 = call "Enqueue Message (Single).vi"("error in (no error)"=w238, "Message Data"="Ready...", "Message"="Update Status", "Message Queue"=w239) -> ("error out"=w245:errorcluster)  [unwired: 6 in, 1 out]
        n75 = call "Enqueue Message (Single).vi"("Priority Message? (F)"=TRUE, "error in (no error)"=w245, "Message"=w242, "Message Queue"=w237) -> ("error out"=w244:errorcluster)  [unwired: 6 in, 1 out]
        n76 = call "Enqueue Message (Single).vi"("error in (no error)"=w244, "Message"=w242, "Message Queue"=w236) -> ("error out"=w243:errorcluster)  [unwired: 7 in, 1 out]
        n77 = call "Enqueue Message (Single).vi"("error in (no error)"=w243, "Message"=w242, "Message Queue"=w235) -> ("error out"=w229:errorcluster)  [unwired: 7 in, 1 out]
        n78 = case shown="Default" w247 {
          selector: w247 -> [_ w249]
          tunnel: [UI_State."Waiting for Stop" ("UI State") w249] -> w246
          frame Default {
          }
          frame "Waiting for Exit" {
          }
        }
        n79 = local write "Logging Status"(FALSE ("Logging Status")) -> ()
      }
      frame "Update Config" {
        n80 = Variant To Data(error in=w256, type="", Variant=w253) -> (data=w252:string, error out=w255:errorcluster)
        n81 = case shown="No Error" w255 {
          selector: w255 -> [w273 w306]
          tunnel: w257 -> [w278 _]
          tunnel: w262 -> [w277 _]
          tunnel: [w276 w306] -> w263
          tunnel: w258 -> [w275 _]
          tunnel: w259 -> [w274 _]
          tunnel: w252 -> [w269 _]
          tunnel: w251 -> [w268 _]
          tunnel: w250 -> [w266 _]
          frame No Error {
            n82 = call "readJsonConfig.vi"("error in"=w273, "jsonConfig"=w269) -> ("error out"=w272:errorcluster, "DAQmx Cluster Out"=w270:T11, "StreamCluster"=w267:T12, "Calibration Configuration Out"=w271:T13)  [unwired: 6 in]
            n83 = case shown="No Error" w272 {
              selector: w272 -> [w295 w305]
              tunnel: w278 -> [w294 _]
              tunnel: w277 -> [w293 _]
              tunnel: w270 -> [w292 _]
              tunnel: [w288 w305] -> w276
              tunnel: w275 -> [w290 _]
              tunnel: w271 -> [w289 _]
              tunnel: w274 -> [w287 _]
              tunnel: w268 -> [w284 _]
              tunnel: w267 -> [w280 _]
              tunnel: w266 -> [w279 _]
              frame No Error {
                w281 = "Update Config"
                n84 = global write "Global 1.vi" "Calibration Configuration Out"(w289) -> ()
                n85 = call "Enqueue Message (Single).vi"("error in (no error)"=w295, "Message Data"=w289, "Message"=w281, "Message Queue"=w294) -> ("error out"=w286:errorcluster)  [unwired: 6 in, 1 out]
                n86 = call "Enqueue Message (Single).vi"("error in (no error)"=w286, "Message Data"=w292, "Message"=w281, "Message Queue"=w293) -> ("error out"=w291:errorcluster)  [unwired: 6 in, 1 out]
                n87 = call "Enqueue Message (Single).vi"("error in (no error)"=w291, "Message Data"=w289, "Message"=w281, "Message Queue"=w290) -> ("error out"=w285:errorcluster)  [unwired: 6 in, 1 out]
                n88 = call "Enqueue Message (Single).vi"("error in (no error)"=w285, "Message Data"=w280, "Message"=w281, "Message Queue"=w284) -> ("error out"=w282:errorcluster)  [unwired: 6 in, 1 out]
                n89 = call "Enqueue Message (Single).vi"("error in (no error)"=w282, "Message Data"=w280, "Message"=w281, "Message Queue"=w279) -> ("error out"=w283:errorcluster)  [unwired: 6 in, 1 out]
                n90 = case shown="No Error" w283 {
                  selector: w283 -> [w302 w304]
                  tunnel: [w298 w304] -> w288
                  tunnel: w287 -> [w303 _]
                  frame No Error {
                    n91 = call "Enqueue Message (Single).vi"("error in (no error)"=w302, "Message Data"="Config file read...Ready..." ("Message"), "Message"="Update Status", "Message Queue"=w303) -> ("error out"=w299:errorcluster, "dup Message Queue"=w297:refnum<queue>)  [unwired: 6 in]
                    n92 = call "Enqueue Message (Single).vi"("error in (no error)"=w299, "Message"="Start", "Message Queue"=w297) -> ("error out"=w298:errorcluster)  [unwired: 7 in, 1 out]
                  }
                  frame Error {
                  }
                }
              }
              frame Error {
              }
            }
          }
          frame Error {
          }
        }
      }
      frame "Sequence Load" {
        n93 = call "Sequence Dialog.vi"("error in (no error)"=w313, "Sequence Conditions In"=w310) -> ("error out"=w312:errorcluster, "Cancelled?"=w311:bool, "Sequence Conditions Out"=w317:T3)  [unwired: 6 in, 1 out]
        n94 = case shown="False" w311 {
          tunnel: [w321 w322] -> w315
          tunnel: w312 -> [w320 w322]
          tunnel: w314 -> [w319 _]
          frame False {
            n95 = call "Enqueue Message (Single).vi"("error in (no error)"=w320, "Message"="Broadcast Sequence", "Message Queue"=w319) -> ("error out"=w321:errorcluster)  [unwired: 7 in, 1 out]
          }
          frame True {
          }
        }
      }
      frame "ASequence Load" {
        n96 = call "Sequence Dialog.vi"("error in (no error)"=w330, "Sequence Conditions In"=w326) -> ("error out"=w329:errorcluster, "Cancelled?"=w328:bool, "Sequence Conditions Out"=w325:T3)  [unwired: 6 in, 1 out]
        n97 = case shown="False" w328 {
          tunnel: [w337 w338] -> w332
          tunnel: w329 -> [w336 w338]
          tunnel: w331 -> [w335 _]
          frame False {
            n98 = call "Enqueue Message (Single).vi"("error in (no error)"=w336, "Message"="Broadcast Sequence", "Message Queue"=w335) -> ("error out"=w337:errorcluster)  [unwired: 7 in, 1 out]
          }
          frame True {
          }
        }
      }
      frame "Broadcast Sequence" {
        n99 = call "Enqueue Message (Single).vi"("error in (no error)"=w346, "Message Data"=w348, "Message"="Update Sequence", "Message Queue"=w340) -> ("error out"=w343:errorcluster, "dup Message Queue"=w341:refnum<queue>)  [unwired: 6 in]
        n100 = call "Enqueue Message (Single).vi"("error in (no error)"=w343, "Message Data"=w344, "Message"="Update AbortSequence", "Message Queue"=w341) -> ("error out"=w342:errorcluster)  [unwired: 6 in, 1 out]
      }
      frame "Launch Aborts" {
        n101 = call "Aborts Dialog.vi"("error in (no error)"=w357, "Abort Parameters In"=w355) -> ("error out"=w356:errorcluster, "Cancelled?"=w353:bool, "Abort Parameters Out"=w354:T5)  [unwired: 6 in, 1 out]
        n102 = case shown="False" w353 {
          tunnel: [w365 w366] -> w359
          tunnel: w356 -> [w364 w366]
          tunnel: w360 -> [w363 _]
          frame False {
            n103 = call "Enqueue Message (Single).vi"("error in (no error)"=w364, "Message"="Broadcast Aborts", "Message Queue"=w363) -> ("error out"=w365:errorcluster)  [unwired: 7 in, 1 out]
          }
          frame True {
          }
        }
      }
      frame "Broadcast Aborts" {
        n104 = call "Enqueue Message (Single).vi"("error in (no error)"=w373, "Message Data"=w369, "Message"="Update Aborts", "Message Queue"=w372) -> ("error out"=w370:errorcluster)  [unwired: 6 in, 1 out]
      }
      frame "Launch BBControl" {
        n105 = call "BBControl Dialog.vi"("error in (no error)"=w382, "BBCont Parameters In"=w378) -> ("error out"=w381:errorcluster, "Cancelled?"=w380:bool, "BBCont Parameters Out"=w376:T2)  [unwired: 6 in, 1 out]
        n106 = case shown="False" w380 {
          tunnel: [w390 w391] -> w384
          tunnel: w381 -> [w389 w391]
          tunnel: w385 -> [w388 _]
          frame False {
            n107 = call "Enqueue Message (Single).vi"("error in (no error)"=w389, "Message"="Broadcast BBControl", "Message Queue"=w388) -> ("error out"=w390:errorcluster)  [unwired: 7 in, 1 out]
          }
          frame True {
          }
        }
      }
      frame "Broadcast BBControl" {
        n108 = call "Enqueue Message (Single).vi"("error in (no error)"=w398, "Message Data"=w393, "Message"="Update BBControl", "Message Queue"=w392) -> ("error out"=w396:errorcluster)  [unwired: 6 in, 1 out]
      }
      frame "Load File Name" {
        n109 = call "Enqueue Message (Single).vi"("error in (no error)"=w410, "Message Data"=w404, "Message"=w403, "Message Queue"=w405) -> ("error out"=w406:errorcluster)  [unwired: 6 in, 1 out]
      }
      frame "System Monitor" {
        n110 = call "System Monitor.vi"("error in (no error)"=w414) -> ("error out"=w413:errorcluster)  [unwired: 10 in]
      }
      frame "Control Monitor" {
        n111 = vi-ref "Control Monitor.vi"() -> (w422:refnum<vi>)
        n112 = invoke class="VI" method="FP.Open"(reference=w422, error in=w421) -> (error out=w420:errorcluster)  [unwired: 3 in, 4 out]
      }
      frame "Soft Controller" {
        n113 = vi-ref "Channel Inputs.vi"() -> (w430:refnum<vi>)
        n114 = invoke class="VI" method="FP.Open"(reference=w430, error in=w429) -> (error out=w428:errorcluster)  [unwired: 3 in, 4 out]
      }
      frame "Graph Display" {
        n115 = vi-ref "GraphDisplay.vi"() -> (w442:refnum<vi>)
        n116 = property class="VI Interface Type 0"(reference=w442) -> ("Name"=w441:string)  [unwired: 1 in, 2 out]
        n117 = Open VI Reference(type specifier VI Refnum (for type only)=w442, vi path=w441, options=192, error in (no error)=w439) -> (vi reference=w444:refnum<vi>, error out=w443:errorcluster)  [unwired: 2 in]
        n118 = call-by-ref "Start Asynchronous Call"(reference=w444, error in=w443, "notifier out"=w435) -> (reference out=w436:refnum<vi>, error out=w438:errorcluster)  [unwired: 3 in]
        n119 = Close Reference(reference=w436, error in (no error)=w438) -> (error out=w437:errorcluster)
      }
      frame "Error" {
        n120 = Variant To Data(error in=w457, type=errorcluster {"status"=FALSE, "code"=0, "source"=""} ("error out"), Variant=w461) -> (data=w453:errorcluster)  [unwired: 1 out]
        n121 = call <vilib>:"Simple Error Handler.vi"("error in (no error)"=w453) -> ()  [unwired: 4 in, 5 out]
        n122 = Unbundle By Name(w453) -> ("source"=w452:string)
        n123 = call "Enqueue Message (Single).vi"("Message Data"=w452, "Message"="Send Error", "Message Queue"=w450) -> ("error out"=w451:errorcluster)  [unwired: 7 in, 1 out]
        n124 = Merge Errors(w451) -> (w462:errorcluster)
      }
      frame "Confirm Quit" {
        n125 = case shown="\"Acquiring\"" w471 {
          selector: w471 -> [_ w478]
          tunnel: [UI_State."Idle" ("UI State") w479] -> w470
          tunnel: w469 -> [w476 w481]
          tunnel: w468 -> [w475 w482]
          tunnel: [w473 w480] -> w467
          frame Default {
            n126 = call "Enqueue Message (Single).vi"("Priority Message? (F)"=TRUE, "error in (no error)"=w476, "Message"="Leave", "Message Queue"=w475) -> ("error out"=w473:errorcluster)  [unwired: 6 in, 1 out]
          }
          frame "Acquiring" {
            n127 = Two Button Dialog(message="Are you sure you want to quit?", 1:"No" ("F button name (\"Cancel\")"), 2:"Yes" ("T button name (\"OK\")")) -> (T button?=w483:bool)
            n128 = case shown="False" w483 {
              tunnel: w482 -> [_ w492]
              tunnel: w481 -> [w488 w491]
              tunnel: [w488 w490] -> w480
              tunnel: [w487 UI_State."Waiting for Exit" ("UI State")] -> w479
              tunnel: w478 -> [w487 _]
              frame False {
              }
              frame True {
                n129 = call "Enqueue Message (Single).vi"("error in (no error)"=w491, "Message"="Stop", "Message Queue"=w492) -> ("error out"=w490:errorcluster)  [unwired: 7 in, 1 out]
              }
            }
          }
        }
      }
      frame "Leave" {
        w494 = "Leave"
        w505 = TRUE
        n130 = Release Notifier(notifier=w504, error in (no error)=w499) -> (error out=w498:errorcluster)  [unwired: 1 in, 2 out]
        n131 = Release Queue(queue=w508, error in (no error)=w499) -> (error out=w502:errorcluster)  [unwired: 1 in, 2 out]
        n132 = Release Queue(queue=w503, error in (no error)=w499) -> (error out=w501:errorcluster)  [unwired: 1 in, 2 out]
        n133 = call "Enqueue Message (Single).vi"("Priority Message? (F)"=w505, "Message"=w494, "Message Queue"=w513) -> ()  [unwired: 7 in, 2 out]
        n134 = Merge Errors(w502, w501, w498) -> (w500:errorcluster)
        n135 = call "Enqueue Message (Single).vi"("Priority Message? (F)"=w505, "Message"=w494, "Message Queue"=w512) -> ()  [unwired: 7 in, 2 out]
        n136 = call "Enqueue Message (Single).vi"("Priority Message? (F)"=w505, "Message"=w494, "Message Queue"=w511) -> ()  [unwired: 7 in, 2 out]
        n137 = call "Enqueue Message (Single).vi"("Priority Message? (F)"=w505, "Message"=w494, "Message Queue"=w509) -> ()  [unwired: 7 in, 2 out]
        n138 = call "Enqueue Message (Single).vi"("Priority Message? (F)"=w505, "Message"=w494, "Message Queue"=w510) -> ()  [unwired: 7 in, 2 out]
        n139 = call "Fire User Event - Stop.vi"("User Event - Stop"=w514) -> ("error out"=w506:errorcluster)  [unwired: 10 in]
        n140 = call "Enqueue Message (Single).vi"("Message"=w494, "Message Queue"=w495) -> ()  [unwired: 8 in, 2 out]
        n141 = Merge Errors(w506, w500) -> (w507:errorcluster)
      }
      frame Default {
        n142 = xnode "Error Ring"("parameter 0"=w523) -> ("error out"=w524:errorcluster)
      }
    }
    n143 = call "Error Handler - Message Handling Loop.vi"("error in (no error)"=w114, "Message Queue"=w118) -> ("dup error in"=w126:errorcluster)  [unwired: 8 in, 1 out]
  }
  n144 = Tick Count (ms)() -> (millisecond timer value=w15:u32)
  n145 = while {
    tunnel: w4 -> [w547]
    shift-right: [w544] -> _
    shift-left: w15 -> [w548]
    tunnel: w6 -> [w542]
    tunnel: w13 -> [w541]
    tunnel: w4 -> [w540]
    tunnel: w3 -> [w536]
    stop <- w546 stop-if-true
    # "Display Loop"
    n146 = Tick Count (ms)() -> (millisecond timer value=w544:u32)
    n147 = Wait on Notification(notifier=w547, ignore previous (F)=TRUE) -> (notification=w538:T6, error out=w546:errorcluster)  [unwired: 2 in, 2 out]
    n148 = Get Notifier Status(notifier=w536) -> (current notification=w534:T4, error out=w535:errorcluster)  [unwired: 1 in, 3 out]
    n149 = Get Date/Time In Seconds() -> (seconds since 1Jan1904=→"Timestamp":timestamp)
    n150 = Subtract(x=w544, y=w548) -> (x-y=w543:u32)
    "Display-Loop Iteration Clock (ms)" <- w543
    n151 = Unbundle By Name(w546) -> ("status"=w545:bool)
    n152 = Wait (ms)(milliseconds to wait=u32 100) -> ()  [unwired: 1 out]
    n153 = call <vilib>:"Clear Errors.vi"("error in (no error)"=w535) -> ()  [unwired: 5 in, 2 out]
    n154 = Not(x=w545) -> (.not. x?=w533:bool)
    n155 = case shown="True" w533 {
      tunnel: w538 -> [_ _]
      tunnel: w543 -> [_ _]
      tunnel: w542 -> [_ w583]
      tunnel: w541 -> [_ w582]
      tunnel: w540 -> [_ w581]
      tunnel: w534 -> [_ w580]
      frame False {
      }
      frame True {
        n156 = Unbundle By Name(w580) -> ("Data Out"=w554:cluster{"DO":bool[], "Module Number":string}[])
        n157 = Unbundle By Name(w583) -> ("UI"=w576:refnum<queue>, "Acquisition"=w575:refnum<queue>, "Logging"=w574:refnum<queue>, "Controls"=w573:refnum<queue>, "Sequence"=w571:refnum<queue>, "Aborts"=w572:refnum<queue>, "Network Streams"=w555:refnum<queue>)
        n158 = Index Array(array=w554, index=0) -> (element=w552:cluster{"DO":bool[], "Module Number":string})
        n159 = call <vilib>:"Get Memory Status.vi"() -> ("free physical memory"=→"Free Physical Memory":u64, "memory allocated for LabVIEW"=→"Memory Allocated For LabVIEW":u64, "total physical memory"=→"Total Physical Memory":u64)  [unwired: 8 in, 1 out]
        n160 = Unbundle(w552) -> ("DO"=w550:bool[])  [unwired: 1 out]
        n161 = for {
          tunnel: w550 -> [w585] mode=indexing
          tunnel: [w584] -> w551 mode=indexing
          n162 = Boolean To (0,1)(Boolean=w585) -> (0, 1=w584:i16)
        }
        "Waveform Chart" <- w551
        n163 = Get Queue Status(queue=w582) -> (# elements in queue=→"Unprocessed Data":i32)  [unwired: 2 in, 7 out]
        n164 = Get Queue Status(queue=w576) -> (# elements in queue=→"UI Elements":i32)  [unwired: 2 in, 7 out]
        n165 = Get Queue Status(queue=w575) -> (# elements in queue=→"Acquisition Elements":i32)  [unwired: 2 in, 7 out]
        n166 = Get Queue Status(queue=w574) -> (# elements in queue=→"Logging Elements":i32)  [unwired: 2 in, 7 out]
        n167 = Get Queue Status(queue=w573) -> (# elements in queue=→"Controls Elements":i32)  [unwired: 2 in, 7 out]
        n168 = Get Queue Status(queue=w571) -> (# elements in queue=→"Sequence Elements":i32)  [unwired: 2 in, 7 out]
        n169 = Get Queue Status(queue=w572) -> (# elements in queue=→"Aborts Elements":i32)  [unwired: 2 in, 7 out]
        n170 = Get Queue Status(queue=w555) -> (# elements in queue=→"NetworkStream Elements":i32)  [unwired: 2 in, 7 out]
        n171 = Get Notifier Status(notifier=w581) -> (# waiting=→"Processed Data":i32)  [unwired: 1 in, 4 out]
        n172 = global read "Globals.vi" "Processing_Logging Iteration Clock"() -> (→"Processing_Logging Iteration Clock":u32)
        n173 = global read "Globals.vi" "Sequencing Iteration Clock"() -> (→"Sequencing Iteration Clock":u32)
        n174 = global read "Globals.vi" "Acquisition Iteration Clock"() -> (→"Acquisition Iteration Clock":u32)
        n175 = global read "Globals.vi" "Controls Iteration Clock"() -> (→"Controls Iteration Clock":u32)
        n176 = global read "Globals.vi" "Aborts Iteration Clock"() -> (→"Aborts Iteration Clock":u32)
        n177 = global read "Globals.vi" "Network Stream Clock"() -> (→"Network Stream Clock":u32)
      }
    }
  }
  n178 = Unregister For Events(event registration refnum=w36, error in=w37) -> (error out=w34:errorcluster)
  n179 = Merge Errors(w34, w33, w24, w23, w21, w9, w18, w8) -> (w22:errorcluster)
  n180 = call "Destroy User Event - Stop.vi"("error in (no error)"=w22, "User Event - Stop"=w28) -> ("error out"=w14:errorcluster)  [unwired: 9 in]
  n181 = call <vilib>:"Simple Error Handler.vi"("error in (no error)"=w14) -> ()  [unwired: 4 in, 5 out]
